vi "Close.vi"(8 "Error In":errorcluster, 11 "Adept Config":T1) -> (0 "Error Out":errorcluster)   [LabVIEW 2011, in "LVH-Adept.lvlib"]
uses:
  <vilib>/LabVIEW Hacker/Adept/LVH-Adept.lvlib
  <vilib>/LabVIEW Hacker/Adept/Private/Type Defs/Device Config.ctl
  <vilib>/LabVIEW Hacker/Adept/Private/Type Defs/Status.ctl
  <vilib>/LabVIEW Hacker/Adept/Private/DMGR/DMGR.lvlib
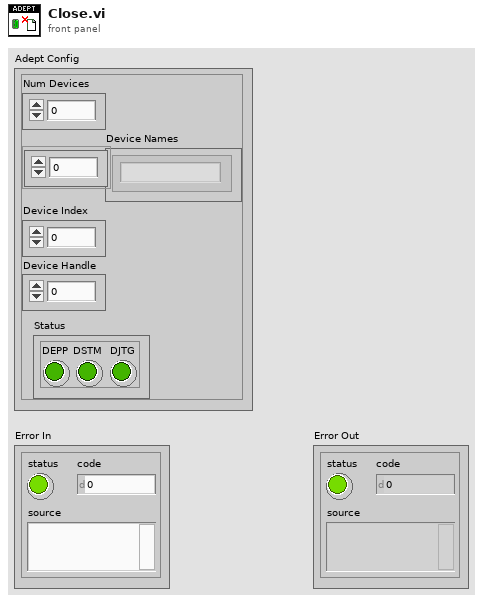
[diagram p1: front panel]
types:
  T1 = typedef "LVH-Adept.lvlib/Device Config.ctl" = cluster{"Num Devices":i32, "Device Names":string[], "Device Index":u16, "Device Handle":u32, "Status":T2}
  T2 = typedef "LVH-Adept.lvlib/Status.ctl" = cluster{"DEPP":bool, "DSTM":bool, "DJTG":bool}
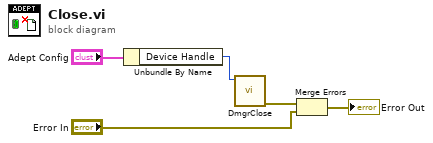
[diagram p0: block diagram]
diagram:
  n1 = Unbundle By Name("Adept Config") -> ("Device Handle"=w4:u32)
  n2 = call <vilib>:"DmgrClose.vi"("hif"=w4) -> ("Error Out"=w3:errorcluster)  [unwired: 10 in]
  n3 = Merge Errors(w3, "Error In") -> (→"Error Out":errorcluster)
